vi "show-hide incdec.vi"(6 "Show?":bool, 8 "error in":errorcluster, 9 "SelList[]":refnum<vi>[](array[refnum])) -> (0 "error out":errorcluster, 1 "SelList[] out":refnum<vi>[](array[refnum]))   [LabVIEW 2012, in "Align and Distribute.lvlib"]
doc: "This VI will show or hide all Inc/Dec buttons in the selection. Errors won't make it out."
uses:
  Align and Distribute.lvlib
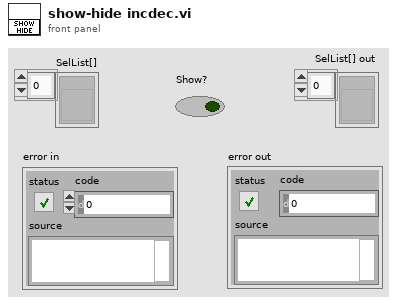
[diagram p1: front panel]
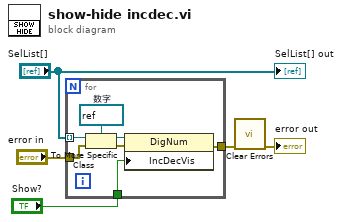
[diagram p0: block diagram]
diagram:
  n1 = for {
    tunnel: "SelList[]" -> [w12] mode=indexing
    tunnel: [w8] -> w4
    tunnel: "error in" -> [w7]
    tunnel: "Show?" -> [w6]
    w10 = refnum<vi> refnum  # 数字
    n2 = To More Specific Class(target class=w10, reference=w12, error in=w7) -> (specific class reference=w11:refnum<vi>, error out=w9:errorcluster)
    n3 = property class="DigNum"(reference=w11, error in=w9, "IncDecVis"=w6) -> (error out=w8:errorcluster)  [unwired: 1 out]
  }
  n4 = call <vilib>:"Clear Errors.vi"("error in (no error)"=w4) -> ("error out"=→"error out":errorcluster)  [unwired: 6 in]
  "SelList[] out" <- "SelList[]"
